vi "dosing control-v2.vi"() -> ()   [LabVIEW 2012]
uses:
  <vilib>/DAQmx/read.llb/DAQmx Read (Analog 1D Wfm NChan NSamp).vi
  <vilib>/DAQmx/create/channels.llb/DAQmx Create Channel (AI-Voltage-Basic).vi
  <vilib>/DAQmx/configure/timing.llb/DAQmx Timing (Sample Clock).vi
  <vilib>/DAQmx/miscellaneous.llb/DAQmx Fill In Error Info.vi
panel:
  in  "Low Volt":dbl
  in  "High Volt":dbl=10.0
  in  "High T":dbl=800.0
  in  "Low T":dbl=300.0
  out "Tempreture":dbl format="%.1f"
  out "Pressure":dbl format="%.2f"
  out "Sample Tempreture":dbl(graph)
  in  "?":bool
  out "Overdosing":bool
  in  "Dosing Limit":dbl=20.0 format="%.2f"
  in  "Base Pressure":dbl=6.47 format="%.2f"
  out "Pressure":dbl(graph)
  out "Oxygen (L)":dbl format="%.1f"
  in  "Upper Pressure Limit":dbl=10.0 format="%.2f"
  in  "?":bool
  # "Pressure"
  # "Temperature"
  # "Langmuir"
  # "stop"
  # "start"
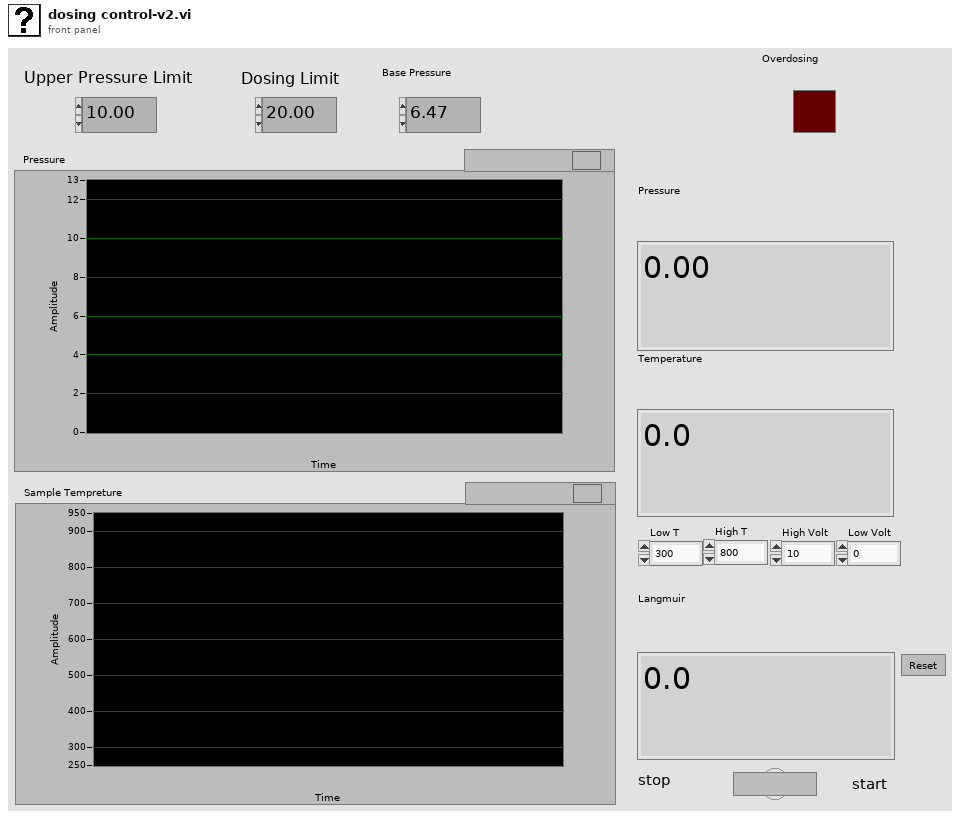
[diagram p1: front panel]
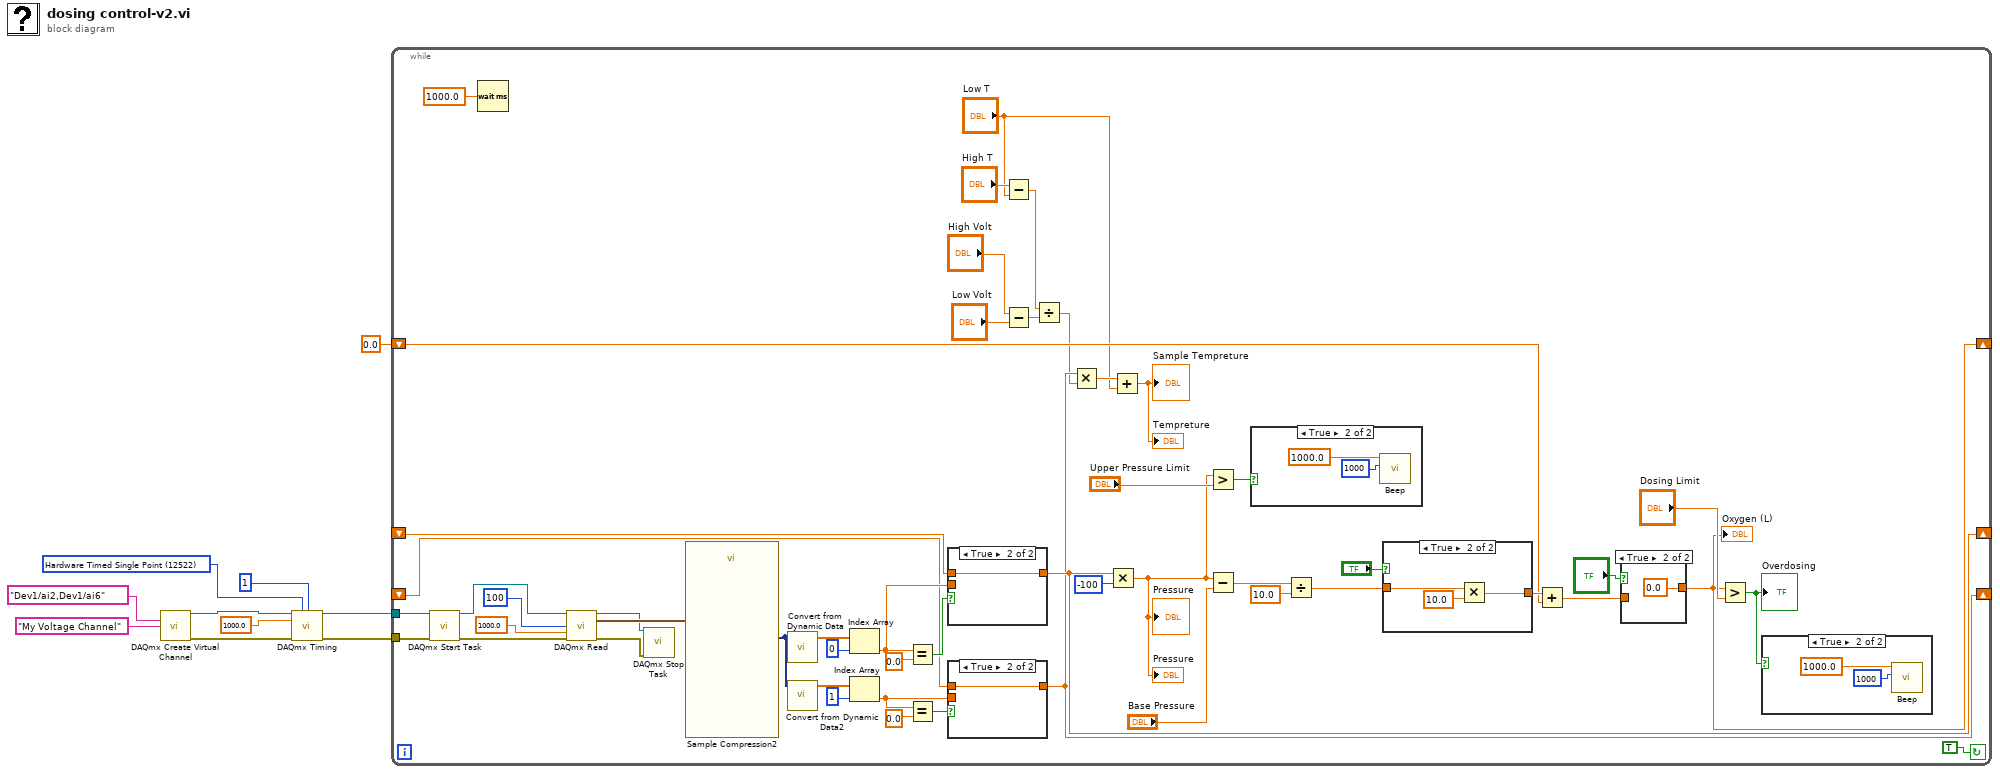
[diagram p0: block diagram]
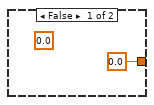
[diagram p6: hidden frame]
diagram:
  w6 = 12522 items=["Finite Samples"=10178, "Continuous Samples"=10123, "Hardware Timed Single Point"=12522] ("sample mode")
  n1 = call-poly <vilib>:"DAQmx Create Virtual Channel.vi"("physical channels"=tag "Dev1/ai2,Dev1/ai6" ("Input Channels"), "name to assign"="My Voltage Channel") -> ("task out"=w5:refnum<k21>, "error out"=w9:errorcluster)  [unwired: 12 in]
  n2 = call-poly <vilib>:"DAQmx Timing.vi"("task/channels in"=w5, "sample mode"=w6, "samples per channel"=1, "rate"=1000.0, "error in"=w9) -> ("task out"=w2:refnum<k21>, "error out"=w1:errorcluster)  [unwired: 9 in]
  n3 = while {
    shift-left: 0.0 -> [w49]
    shift-right: [w47] -> _
    shift-right: [w33] -> _
    shift-left: _ -> [w32]
    shift-right: [w28] -> _
    shift-left: _ -> [w27]
    tunnel: w2 -> [w16]
    tunnel: w1 -> [w14]
    stop <- TRUE continue-if-true
    n4 = call <vilib>:"DAQmx Start Task.vi"("task/channels in"=w16, "error in"=w14) -> ("task out"=w15:refnum<k21>, "error out"=w13:errorcluster)  [unwired: 12 in]
    n5 = Wait (ms)(milliseconds to wait=1000.0 ("y")) -> ()  [unwired: 1 out]
    n6 = call-poly <vilib>:"DAQmx Read.vi"("task/channels in"=w15, "number of samples per channel"=100 ("number of samples"), "timeout"=1000.0 ("rate"), "error in"=w13) -> ("task out"=w12:refnum<k21>, "data"=w17:waveform(dbl)[], "error out"=w11:errorcluster)  [unwired: 9 in]
    n7 = call <vilib>:"DAQmx Stop Task.vi"("task/channels in"=w12, "error in"=w11) -> ()  [unwired: 12 in, 2 out]
    n8 = call "Sample Compression2"("Signals"=w17) -> ("Mean"=w39:dynamicdata)  [unwired: 8 in, 2 out]
    n9 = call "Convert from Dynamic Data"("Dynamic Data Type"=w39) -> ("Array"=w43:dbl[])  [unwired: 3 in]
    n10 = call "Convert from Dynamic Data2"("Dynamic Data Type"=w39) -> ("Array"=w41:dbl[])  [unwired: 3 in]
    n11 = Index Array(array=w43, index=0) -> (element=w34:dbl)
    n12 = Index Array(array=w41, index=1) -> (element=w29:dbl)
    n13 = Equal?(x=w34, y=0.0) -> (x = y?=w35:bool)
    n14 = Equal?(x=w29, y=0.0) -> (x = y?=w30:bool)
    n15 = case shown="True" w35 {
      tunnel: w34 -> [w64 _]
      tunnel: [w64 w65] -> w33
      tunnel: w32 -> [_ w65]
      frame False {
      }
      frame True {
      }
    }
    n16 = case shown="True" w30 {
      tunnel: w29 -> [w62 _]
      tunnel: [w62 w63] -> w28
      tunnel: w27 -> [_ w63]
      frame False {
      }
      frame True {
      }
    }
    n17 = Subtract(x="High T", y="Low T") -> (x-y=w22:dbl)
    n18 = Subtract(x="High Volt", y="Low Volt") -> (x-y=w21:dbl)
    n19 = Divide(x=w22, y=w21) -> (x/y=w20:dbl)
    n20 = Multiply(x=w28, y=w20) -> (x*y=w44:dbl)
    n21 = Multiply(x=w33, y=-100) -> (x*y=w38:dbl)
    "Pressure" <- w38
    "Pressure" <- w38
    n22 = Add(x=w44, y="Low T") -> (x+y=→"Sample Tempreture" →"Tempreture":dbl)
    n23 = Greater?(x=w38, y="Upper Pressure Limit") -> (0:w60:bool)
    n24 = Subtract(x=w38, y="Base Pressure") -> (x-y=w53:dbl)
    n25 = case shown="True" w60 {
      frame False {
      }
      frame True {
        n26 = call <vilib>:"Beep.vi"("duration (msec)"=i16 1000 ("duration (msec) - ignored"), "frequency (Hz)"=1000.0 ("frequency (Hz) - ignored")) -> ()  [unwired: 10 in]
      }
    }
    n27 = Divide(x=w53, y=10.0) -> (x/y=w57:dbl)
    n28 = case shown="True" "?" {
      tunnel: [0.0 w71] -> w50
      tunnel: w57 -> [_ w73]
      frame False {
        (unwired) 0.0
      }
      frame True {
        n29 = Multiply(x=w73, y=10.0) -> (x*y=w71:dbl)
      }
    }
    n30 = Add(x=w50, y=w49) -> (x+y=w48:dbl)
    n31 = case shown="True" "?" {
      tunnel: w48 -> [w66 _]
      tunnel: [w66 0.0 ("y")] -> w47
      frame False {
      }
      frame True {
      }
    }
    "Oxygen (L)" <- w47
    n32 = Greater?(x=w47, y="Dosing Limit") -> (0:w51:bool)
    "Overdosing" <- w51
    n33 = case shown="True" w51 {
      frame False {
      }
      frame True {
        n34 = call <vilib>:"Beep.vi"("duration (msec)"=i16 1000 ("duration (msec) - ignored"), "frequency (Hz)"=1000.0 ("frequency (Hz) - ignored")) -> ()  [unwired: 10 in]
      }
    }
  }
